vi "general_measurement_HT.vi"(9 "Measurement Data":dbl[](array[numeric]), 10 "Array 4":dbl[](array[numeric]), 11 "Array 3":dbl[](array[numeric])) -> (1 "Measurement":T1, 2 "Array":dbl[](array[numeric]), 3 "Array 2":dbl[](array[numeric]), 4 "Array 5":dbl[](array[numeric]), 5 "Seebeck coefficient":cluster{"Y":dbl[], "Y":dbl[]}[](graph))   [LabVIEW 2011]
uses:
  <vilib>/express/express arith-compare/Formula/XNode/ExpressFormulaBlockNode.xnode
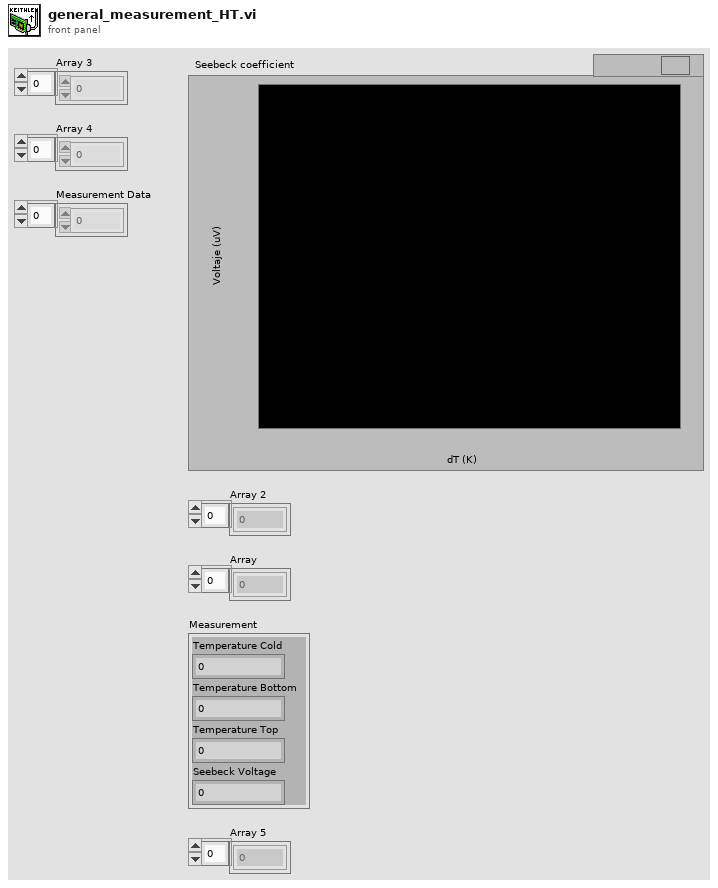
[diagram p1: front panel]
types:
  T1 = cluster{"Temperature Cold":dbl, "Temperature Bottom":dbl, "Temperature Top":dbl, "Seebeck Voltage":dbl}
  T2 = cluster{"Measurement Data[0]":dbl, "Measurement Data[1]":dbl, "Measurement Data[2]":dbl, "Measurement Data[3]":dbl, "Measurement Data[4]":dbl, "Measurement Data[5]":dbl, "Measurement Data[6]":dbl, "Measurement Data[7]":dbl, "Measurement Data[8]":dbl}
  T3 = cluster{"Result":dbl, "Result":dbl, "Result":dbl, "Measurement Data[3]":dbl}
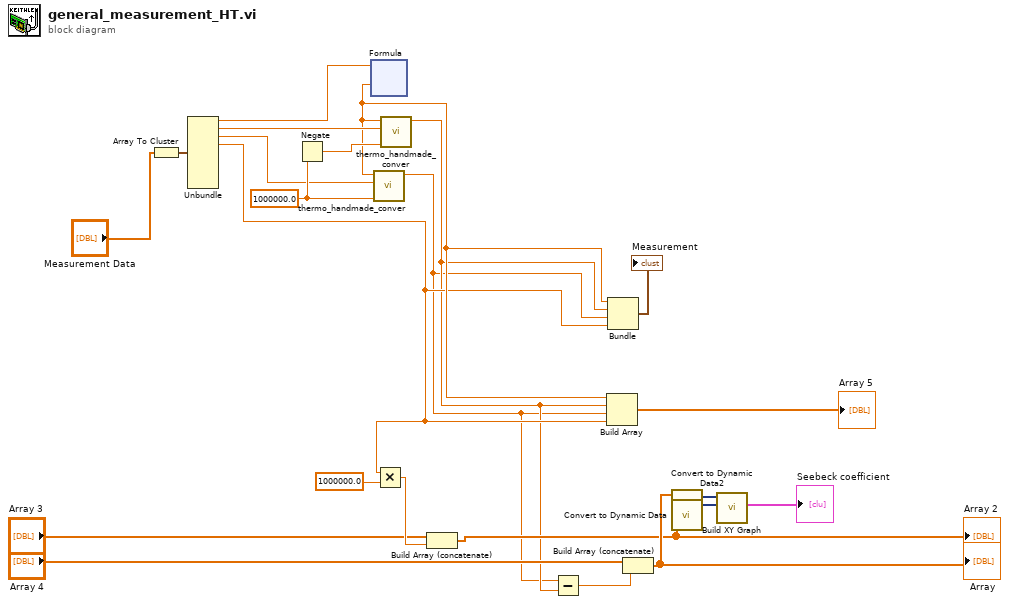
[diagram p0: block diagram]
diagram:
  w23 = 1000000.0 ("y")
  n1 = Array To Cluster(array="Measurement Data") -> (cluster=w6:T2)
  n2 = Unbundle(w6) -> ("Measurement Data[0]"=w12:dbl, "Measurement Data[1]"=w9:dbl, "Measurement Data[2]"=w10:dbl, "Measurement Data[3]"=w3:dbl)  [unwired: 5 out]
  n3 = Negate(x=w23) -> (-x=w13:dbl)
  n4 = xnode ("Formula")("R"=w12) -> ("Result"=w5:dbl)  [unwired: 1 in, 1 out]
  n5 = call "thermo_handmade_conver.vi"("y"=w23, "Measurement Data[1]"=w10, "Measurement Data[0]"=w5) -> ("Result"=w1:dbl)  [unwired: 8 in]
  n6 = Multiply(x=w3, y=1000000.0 ("x")) -> (x*y=w22:dbl)
  n7 = call "thermo_handmade_conver.vi"("y"=w13, "Measurement Data[1]"=w9, "Measurement Data[0]"=w5) -> ("Result"=w2:dbl)  [unwired: 8 in]
  n8 = Build Array (concatenate)("Array 3", w22) -> (w18:dbl[])
  "Array 2" <- w18
  n9 = Subtract(x=w1, y=w2) -> (x-y=w16:dbl)
  n10 = Build Array(w5, w2, w1, w3) -> (→"Array 5":dbl[])
  n11 = Bundle("Result"=w5, "Result"=w2, "Result"=w1, "Measurement Data[3]"=w3) -> (→"Measurement":T3)  [unwired: 1 in]
  n12 = Build Array (concatenate)("Array 4", w16) -> (w20:dbl[])
  "Array" <- w20
  n13 = call "Convert to Dynamic Data2"("Array"=w20) -> ("Dynamic Data Type"=w21:dynamicdata)  [unwired: 3 in]
  n14 = call "Convert to Dynamic Data"("Array"=w18) -> ("Dynamic Data Type"=w19:dynamicdata)  [unwired: 3 in]
  n15 = call "Build XY Graph"("Y Input"=w19, "X Input"=w21) -> ("XY Graph"=→"Seebeck coefficient":cluster{"Y":dbl[], "Y":dbl[]}[])  [unwired: 3 in, 6 out]
